vi "InitShooter.vi"   [LabVIEW 2019]
uses:
  refnums.vi
  <vilib>/Rock Robotics/WPI/ThirdParty/REV Robotics/SPARK MAX/Typedef/Spark MAX Idle Mode.ctl
  <vilib>/Rock Robotics/WPI/Solenoid/WPI_SolenoidChannel.ctl
  <vilib>/Rock Robotics/WPI/Solenoid/WPI_SolenoidOpenDouble.vi
types:
  T1 = typedef "Spark MAX Idle Mode.ctl" = enum16{"Coast", "Brake"}
  T2 = typedef "WPI_SolenoidChannel.ctl" = enum8{"Solenoid 0", "Solenoid 1", "Solenoid 2", "Solenoid 3", "Solenoid 4", "Solenoid 5", "Solenoid 6", "Solenoid 7", "Invalid"}
  T3 = typedef "WPI_MotorControlDeviceRef.ctl" = cluster{"DeviceStatus":errorcluster, "Type":T4, "PWM":cluster{"PWM Channel":T5, "DeadBand":T6}, "CAN":cluster{"Device Number":u8, "SetOutput VI Ref":variant, "GetOutput VI Ref":variant, "Enable VI Ref":variant, "Disable VI Ref":variant, "Data":variant}, "Invert":bool, "DIO PWM":cluster{"PWM \"Enable\" Channel":T5, "DIOChannel":T7, "PWM Rate":dbl}}
  T4 = typedef "WPI_MotorControlType.ctl" = enum16{"PWM", "CAN", "DIO PWM"}
  T5 = typedef "FPGA_DIOPWMChannel.ctl" = enum8{"PWM 0", "PWM 1", "PWM 2", "PWM 3", "PWM 4", "PWM 5", "PWM 6", "PWM 7", "PWM 8", "PWM 9", "PWM MXP 0", "PWM MXP 1", "PWM MXP 2", "PWM MXP 3", "PWM MXP 4", "PWM MXP 5", "PWM MXP 6", "PWM MXP 7", "PWM MXP 8", "PWM MXP 9", "Invalid"}
  T6 = typedef "WPI_PWMDeadband.ctl" = cluster{"Name":string, "maxPositivePwm":i32, "minPositivePwm":i32, "centerPwm":i32, "maxNegativePwm":i32, "minNegativePwm":i32, "angularRange":u16}
  T7 = typedef "FPGA_DIOChannel.ctl" = enum8{"DIO 0", "DIO 1", "DIO 2", "DIO 3", "DIO 4", "DIO 5", "DIO 6", "DIO 7", "DIO 8", "DIO 9", "DIO MXP 0", "DIO MXP 1", "DIO MXP 2", "DIO MXP 3", "DIO MXP 4", "DIO MXP 5", "DIO MXP 6", "DIO MXP 7", "DIO MXP 8", "DIO MXP 9", "DIO MXP 10", "DIO MXP 11", "DIO MXP 12", "DIO MXP 13", "DIO MXP 14", "DIO MXP 15", "SPI Port CS1", "SPI Port CS2", "SPI Port CS3", "SPI Port MISO", "SPI Port MOSI", "Invalid"}
  T8 = typedef "WPI_SolenoidDevRef.ctl" = cluster{"DevStatus":errorcluster, "Pneumatics Control Module":u8, "Forward Solenoid Channel":T2, "Reverse Solenoid Channel":T2}
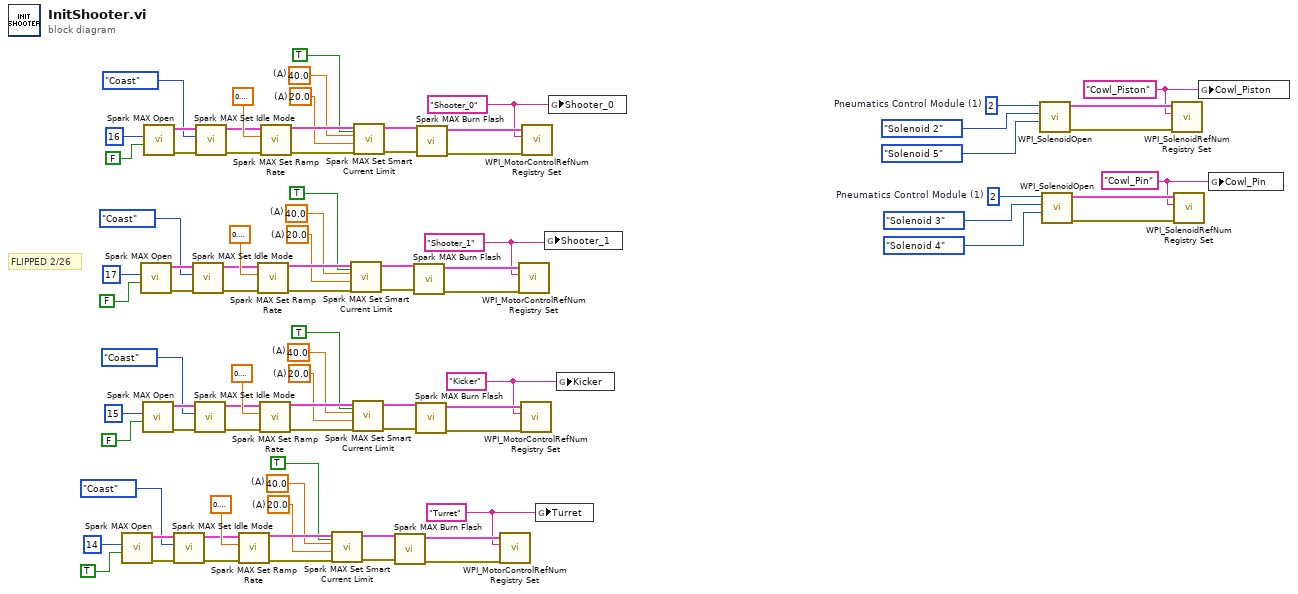
[diagram p0: block diagram]
diagram:
  w8 = 40.0  # (A)
  w7 = 20.0  # (A)
  w4 = "Turret" ("refnum name")
  w19 = "Cowl_Pin" ("refnum name")
  w24 = u8 2  # Pneumatics Control Module (1)
  w25 = "Cowl_Piston" ("refnum name")
  w30 = u8 2  # Pneumatics Control Module (1)
  w38 = 40.0  # (A)
  w37 = 20.0  # (A)
  w34 = "Kicker" ("refnum name")
  w59 = 40.0  # (A)
  w58 = 20.0  # (A)
  w54 = "Shooter_1" ("refnum name")
  w73 = 40.0  # (A)
  w72 = 20.0  # (A)
  w55 = "Shooter_0" ("refnum name")
  # "FLIPPED 2/26"
  n1 = call <vilib>:"Spark MAX Open.vi"("Invert"=TRUE, "Device Number"=u8 14 ("Drive 1R")) -> ("error out"=w15:errorcluster, "MotorControlDeviceRef"=w18:T3)  [unwired: 8 in]
  n2 = call <vilib>:"Spark MAX Open.vi"("Invert"=FALSE, "Device Number"=u8 17 ("Drive 1R")) -> ("error out"=w66:errorcluster, "MotorControlDeviceRef"=w69:T3)  [unwired: 8 in]
  n3 = call <vilib>:"Spark MAX Open.vi"("Invert"=FALSE, "Device Number"=u8 15 ("Drive 1R")) -> ("error out"=w45:errorcluster, "MotorControlDeviceRef"=w48:T3)  [unwired: 8 in]
  n4 = call <vilib>:"Spark MAX Open.vi"("Invert"=FALSE, "Device Number"=u8 16 ("Drive 1R")) -> ("error out"=w80:errorcluster, "MotorControlDeviceRef"=w83:T3)  [unwired: 8 in]
  n5 = call <vilib>:"Spark MAX Set Idle Mode.vi"("error in (no error)"=w15, "Idle Mode"=Spark_MAX_Idle_Mode."Coast", "MotorControlDeviceRef in"=w18) -> ("error out"=w2:errorcluster, "MotorControlDeviceRef out"=w3:T3)  [unwired: 7 in]
  n6 = call <vilib>:"Spark MAX Set Idle Mode.vi"("error in (no error)"=w66, "Idle Mode"=Spark_MAX_Idle_Mode."Coast", "MotorControlDeviceRef in"=w69) -> ("error out"=w52:errorcluster, "MotorControlDeviceRef out"=w53:T3)  [unwired: 7 in]
  n7 = call <vilib>:"Spark MAX Set Idle Mode.vi"("error in (no error)"=w45, "Idle Mode"=Spark_MAX_Idle_Mode."Coast", "MotorControlDeviceRef in"=w48) -> ("error out"=w32:errorcluster, "MotorControlDeviceRef out"=w33:T3)  [unwired: 7 in]
  n8 = call <vilib>:"Spark MAX Set Idle Mode.vi"("error in (no error)"=w80, "Idle Mode"=Spark_MAX_Idle_Mode."Coast", "MotorControlDeviceRef in"=w83) -> ("error out"=w50:errorcluster, "MotorControlDeviceRef out"=w51:T3)  [unwired: 7 in]
  n9 = call <vilib>:"Spark MAX Set Ramp Rate.vi"("error in (no error)"=w2, "Seconds from neutral to full (0)"=sgl 0.2, "MotorControlDeviceRef in"=w3) -> ("error out"=w12:errorcluster, "MotorControlDeviceRef"=w9:T3)  [unwired: 7 in]
  n10 = call <vilib>:"Spark MAX Set Ramp Rate.vi"("error in (no error)"=w52, "Seconds from neutral to full (0)"=sgl 0.2, "MotorControlDeviceRef in"=w53) -> ("error out"=w63:errorcluster, "MotorControlDeviceRef"=w60:T3)  [unwired: 7 in]
  n11 = call <vilib>:"Spark MAX Set Ramp Rate.vi"("error in (no error)"=w32, "Seconds from neutral to full (0)"=sgl 0.2, "MotorControlDeviceRef in"=w33) -> ("error out"=w42:errorcluster, "MotorControlDeviceRef"=w39:T3)  [unwired: 7 in]
  n12 = call <vilib>:"Spark MAX Set Ramp Rate.vi"("error in (no error)"=w50, "Seconds from neutral to full (0)"=sgl 0.2, "MotorControlDeviceRef in"=w51) -> ("error out"=w77:errorcluster, "MotorControlDeviceRef"=w74:T3)  [unwired: 7 in]
  n13 = call <vilib>:"Spark MAX Set Smart Current Limit.vi"("Linearized Limit Enabled (F)"=TRUE, "error in (no error)"=w12, "Free Speed Current Limit (20A)"=w7, "Primay Current Limit (80A)"=w8, "MotorControlDeviceRef in"=w9) -> ("error out"=w11:errorcluster, "MotorControlDeviceRef out"=w10:T3)  [unwired: 5 in]
  n14 = call <vilib>:"Spark MAX Set Smart Current Limit.vi"("Linearized Limit Enabled (F)"=TRUE, "error in (no error)"=w63, "Free Speed Current Limit (20A)"=w58, "Primay Current Limit (80A)"=w59, "MotorControlDeviceRef in"=w60) -> ("error out"=w62:errorcluster, "MotorControlDeviceRef out"=w61:T3)  [unwired: 5 in]
  n15 = call <vilib>:"Spark MAX Set Smart Current Limit.vi"("Linearized Limit Enabled (F)"=TRUE, "error in (no error)"=w42, "Free Speed Current Limit (20A)"=w37, "Primay Current Limit (80A)"=w38, "MotorControlDeviceRef in"=w39) -> ("error out"=w41:errorcluster, "MotorControlDeviceRef out"=w40:T3)  [unwired: 5 in]
  n16 = call <vilib>:"Spark MAX Set Smart Current Limit.vi"("Linearized Limit Enabled (F)"=TRUE, "error in (no error)"=w77, "Free Speed Current Limit (20A)"=w72, "Primay Current Limit (80A)"=w73, "MotorControlDeviceRef in"=w74) -> ("error out"=w76:errorcluster, "MotorControlDeviceRef out"=w75:T3)  [unwired: 5 in]
  n17 = call <vilib>:"Spark MAX Burn Flash.vi"("error in"=w11, "MotorControlDeviceRef"=w10) -> ("error out"=w13:errorcluster, "MotorControlDeviceRef"=w14:T3)  [unwired: 8 in]
  n18 = call <vilib>:"Spark MAX Burn Flash.vi"("error in"=w62, "MotorControlDeviceRef"=w61) -> ("error out"=w64:errorcluster, "MotorControlDeviceRef"=w65:T3)  [unwired: 8 in]
  n19 = call <vilib>:"Spark MAX Burn Flash.vi"("error in"=w41, "MotorControlDeviceRef"=w40) -> ("error out"=w43:errorcluster, "MotorControlDeviceRef"=w44:T3)  [unwired: 8 in]
  n20 = call <vilib>:"Spark MAX Burn Flash.vi"("error in"=w76, "MotorControlDeviceRef"=w75) -> ("error out"=w78:errorcluster, "MotorControlDeviceRef"=w79:T3)  [unwired: 8 in]
  n21 = call <vilib>:"WPI_MotorControlRefNum Registry Set.vi"("error in (no error)"=w13, "refnum name"=w4, "MotorControlDevRef"=w14) -> ()  [unwired: 7 in, 2 out]
  n22 = call <vilib>:"WPI_MotorControlRefNum Registry Set.vi"("error in (no error)"=w64, "refnum name"=w54, "MotorControlDevRef"=w65) -> ()  [unwired: 7 in, 2 out]
  n23 = call <vilib>:"WPI_MotorControlRefNum Registry Set.vi"("error in (no error)"=w43, "refnum name"=w34, "MotorControlDevRef"=w44) -> ()  [unwired: 7 in, 2 out]
  n24 = call <vilib>:"WPI_MotorControlRefNum Registry Set.vi"("error in (no error)"=w78, "refnum name"=w55, "MotorControlDevRef"=w79) -> ()  [unwired: 7 in, 2 out]
  n25 = global write "refnums.vi" "Turret"(w4) -> ()
  n26 = global write "refnums.vi" "Shooter_1"(w54) -> ()
  n27 = global write "refnums.vi" "Shooter_0"(w55) -> ()
  n28 = global write "refnums.vi" "Kicker"(w34) -> ()
  n29 = call-poly <vilib>:"WPI_SolenoidOpen.vi"("Reverse Solenoid Channel"=WPI_SolenoidChannel."Solenoid 5", "Forward Solenoid Channel"=WPI_SolenoidChannel."Solenoid 2", "Pneumatics Control Module (0)"=w30) -> ("error out"=w26:errorcluster, "SolenoidDevRef"=w27:T8)  [unwired: 7 in]
  n30 = call-poly <vilib>:"WPI_SolenoidOpen.vi"("Reverse Solenoid Channel"=WPI_SolenoidChannel."Solenoid 4", "Forward Solenoid Channel"=WPI_SolenoidChannel."Solenoid 3", "Pneumatics Control Module (0)"=w24) -> ("error out"=w20:errorcluster, "SolenoidDevRef"=w21:T8)  [unwired: 7 in]
  n31 = call <vilib>:"WPI_SolenoidRefNum Registry Set.vi"("error in (no error)"=w26, "refnum name"=w25, "SolenoidDevRef"=w27) -> ()  [unwired: 7 in, 2 out]
  n32 = call <vilib>:"WPI_SolenoidRefNum Registry Set.vi"("error in (no error)"=w20, "refnum name"=w19, "SolenoidDevRef"=w21) -> ()  [unwired: 7 in, 2 out]
  n33 = global write "refnums.vi" "Cowl_Piston"(w25) -> ()
  n34 = global write "refnums.vi" "Cowl_Pin"(w19) -> ()
